vi "MSScript_SubVI_ArraySplit.vi"(7 "GetValue? (F)":bool, 11 "VarString in":string) -> (0 "Value Error?":bool, 1 "ArrayVariable out":ext[](array[numeric]), 2 "Is a variable?":bool, 3 "@name":string)   [LabVIEW 2018, in "MSScript.lvclass"]
uses:
  MSScript/MSScript.lvclass
  MSScript/MSScript_Transform_EXTArray.vi
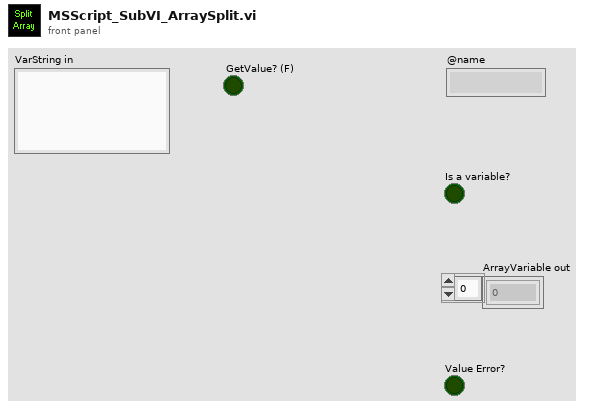
[diagram p1: front panel]
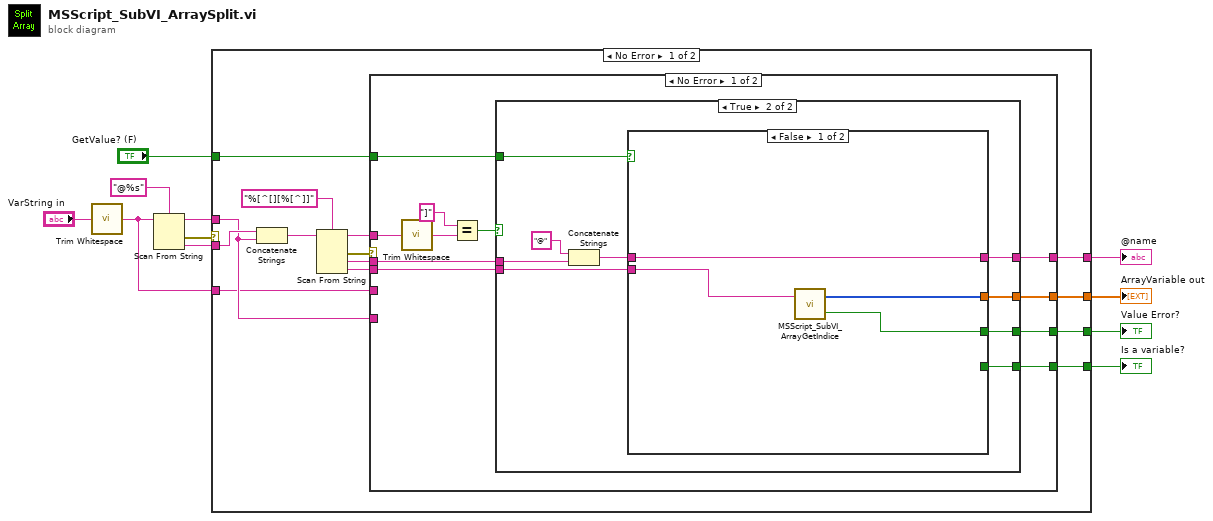
[diagram p0: block diagram]
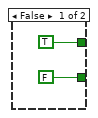
[diagram p2: hidden frame]
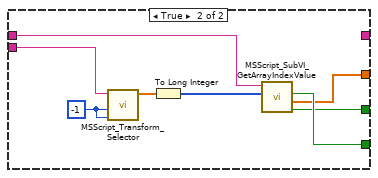
[diagram p3: hidden frame]
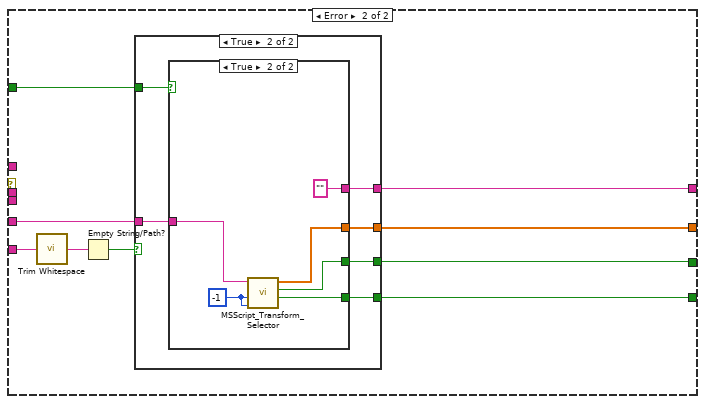
[diagram p4: hidden frame]
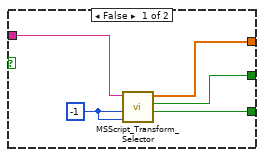
[diagram p5: hidden frame]
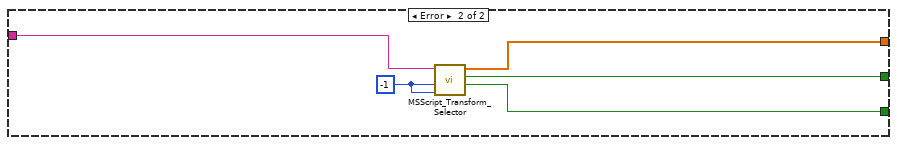
[diagram p7: hidden frame]
diagram:
  n1 = call <vilib>:"Trim Whitespace.vi"("string"="VarString in") -> ("trimmed string"=w5:string)  [unwired: 1 in]
  n2 = Scan From String(format string="@%s", input string=w5) -> (remaining string=w8:string, error out=w9:errorcluster, output 1=w7:string)  [unwired: 3 in, 1 out]
  n3 = case shown="No Error" w9 {
    tunnel: w8 -> [w17 _]
    tunnel: w7 -> [w18 _]
    tunnel: [w19 _] -> w6
    tunnel: w5 -> [w16 w91]
    tunnel: [w13 w89] -> w4
    tunnel: [w15 w88] -> w3
    tunnel: [w14 w87] -> w2
    tunnel: "GetValue? (F)" -> [w12 _]
    frame No Error {
      n4 = Concatenate Strings(w18, w17) -> (w25:string)
      n5 = Scan From String(format string="%[^[][%[^]]", input string=w25) -> (remaining string=w20:string, error out=w23:errorcluster, output 1=w22:string, output 2=w21:string)  [unwired: 4 in, 1 out]
      n6 = case shown="No Error" w23 {
        tunnel: w22 -> [w30 _]
        tunnel: w21 -> [w29 _]
        tunnel: w20 -> [w36 _]
        tunnel: [w27 w68] -> w19
        tunnel: w17 -> [_ w67]
        tunnel: w16 -> [_ w64]
        tunnel: [w28 w60] -> w13
        tunnel: [w32 w63] -> w15
        tunnel: [w31 w62] -> w14
        tunnel: w12 -> [w26 w61]
        frame No Error {
          n7 = call <vilib>:"Trim Whitespace.vi"("string"=w36) -> ("trimmed string"=w35:string)  [unwired: 1 in]
          n8 = Equal?(x="]", y=w35) -> (x = y?=w33:bool)
          n9 = case shown="True" w33 {
            tunnel: [TRUE w40] -> w32
            tunnel: [FALSE w44] -> w31
            tunnel: w30 -> [_ w46]
            tunnel: w29 -> [_ w39]
            tunnel: [_ w42] -> w28
            tunnel: [_ w41] -> w27
            tunnel: w26 -> [_ w45]
            frame False {
            }
            frame True {
              n10 = Concatenate Strings("@" ("string"), w46) -> (w43:string)
              n11 = case shown="False" w45 {
                tunnel: [_ w58] -> w44
                tunnel: w43 -> [w51 w59]
                tunnel: [w50 w56] -> w42
                tunnel: [w51 _] -> w41
                tunnel: [w49 w57] -> w40
                tunnel: w39 -> [w48 w53]
                frame False {
                  n12 = call "MSScript_SubVI_ArrayGetIndice.vi"("indice string in"=w48) -> ("error"=w49:bool, "x:y"=w50:i32[])  [unwired: 1 in]
                }
                frame True {
                  w55 = -1 ("MaxSize")
                  n13 = call-poly "MSScript_Transform_Selector.vi"("MinSize"=w55, "MaxSize"=w55, "check_str"=w53) -> ("Value Output"=w54:ext[])  [unwired: 6 in, 2 out]
                  n14 = To Long Integer(number=w54) -> (32bit integer=w52:i32[])
                  n15 = call "MSScript_SubVI_GetArrayIndexValue.vi"("Index"=w52, "@name"=w59) -> ("Value Error?"=w57:bool, "ArrayVariable out"=w56:ext[], "Is a variable ?"=w58:bool)  [unwired: 7 in]
                }
              }
            }
          }
        }
        frame Error {
          n16 = call <vilib>:"Trim Whitespace.vi"("string"=w67) -> ("trimmed string"=w66:string)  [unwired: 1 in]
          n17 = Empty String/Path?(string/path=w66) -> (empty?=w65:bool)
          n18 = case shown="True" w65 {
            tunnel: [_ w77] -> w68
            tunnel: w64 -> [w73 w79]
            tunnel: [w71 w74] -> w63
            tunnel: [w70 w75] -> w62
            tunnel: w61 -> [_ w78]
            tunnel: [w72 w76] -> w60
            frame False {
              w69 = -1 ("MaxSize")
              n19 = call-poly "MSScript_Transform_Selector.vi"("MinSize"=w69, "MaxSize"=w69, "check_str"=w73) -> ("Is a variable ?"=w70:bool, "Value Error?"=w71:bool, "Value Output"=w72:ext[])  [unwired: 6 in]
            }
            frame True {
              n20 = case shown="True" w78 {
                tunnel: w79 -> [w80 w85]
                tunnel: [w80 ""] -> w77
                tunnel: [_ w84] -> w76
                tunnel: [_ w82] -> w75
                tunnel: [_ w83] -> w74
                frame False {
                }
                frame True {
                  w81 = -1 ("MaxSize")
                  n21 = call-poly "MSScript_Transform_Selector.vi"("MinSize"=w81, "MaxSize"=w81, "check_str"=w85) -> ("Is a variable ?"=w82:bool, "Value Error?"=w83:bool, "Value Output"=w84:ext[])  [unwired: 6 in]
                }
              }
            }
          }
        }
      }
    }
    frame Error {
      w90 = -1 ("MaxSize")
      n22 = call-poly "MSScript_Transform_Selector.vi"("MinSize"=w90, "MaxSize"=w90, "check_str"=w91) -> ("Is a variable ?"=w87:bool, "Value Error?"=w88:bool, "Value Output"=w89:ext[])  [unwired: 6 in]
    }
  }
  "@name" <- w6
  "ArrayVariable out" <- w4
  "Value Error?" <- w3
  "Is a variable?" <- w2
